vi "bring vi to front.vi"(11 "VI Name":string="MacroGUI_MD.vi") -> ()   [LabVIEW 2012]
doc: "SciScan 1.2 160622"
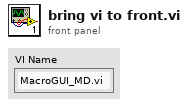
[diagram p1: front panel]
types:
  T1 = enum32{"Invalid", "Standard", "Closed", "Hidden", "Minimized", "Maximized"}
  T2 = enum32{"Invalid", "Default", "Floating", "Floating/Auto-Hide", "Modal"}
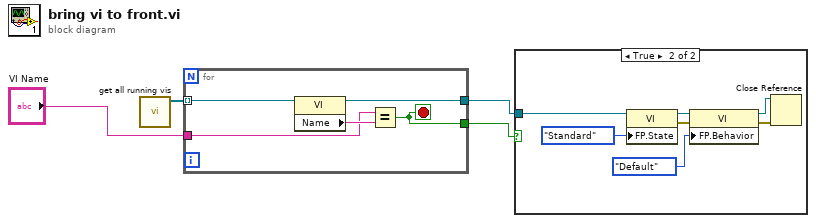
[diagram p0: block diagram]
diagram:
  n1 = call "get all running vis.vi"() -> ("RunningVIRefs"=w4:refnum<vi>[])  [unwired: 11 in]
  n2 = for {
    tunnel: w4 -> [w9] mode=indexing
    tunnel: "VI Name" -> [w7]
    tunnel: [w6] -> w1
    tunnel: [w5] -> w2
    stop <- w6 stop-if-true
    n3 = property class="VI"(reference=w9) -> (reference out=w5:refnum<vi>, "Name"=w8:string)  [unwired: 1 in, 1 out]
    n4 = Equal?(x=w7, y=w8) -> (x = y?=w6:bool)
  }
  n5 = case shown="True" w1 {
    tunnel: w2 -> [_ w15]
    frame False {
    }
    frame True {
      n6 = property class="VI"(reference=w15, "FP.State"=T1."Standard" ("Front Panel Window:State")) -> (reference out=w14:refnum<vi>, error out=w13:errorcluster)  [unwired: 1 in]
      n7 = property class="VI"(reference=w14, error in=w13, "FP.Behavior"=T2."Default" ("Front Panel Window:Behavior")) -> (reference out=w10:refnum<vi>, error out=w11:errorcluster)
      n8 = Close Reference(reference=w10, error in (no error)=w11) -> ()  [unwired: 1 out]
    }
  }
